vi "Init.vi"(4 "Data Queue Names":string[](array[string]), 6 "Data Notifier Names":string[](array[string]), 7 "Name":string, 8 "error in (no error)":errorcluster, 10 "MSS":refnum<class "Measure and Stimulus Subsystems.lvclass">, 11 "Sample PID Light in":refnum<class "Sample PID Light.lvclass">) -> (0 "error out":errorcluster, 3 "Sample PID Light out":refnum<class "Sample PID Light.lvclass">)   [LabVIEW 2023, in "Sample PID Light.lvclass"]
uses:
  Sample PID Light.lvclass
  Measure and Stimulus Subsystems/Measure and Stimulus Subsystems.lvclass
  Task/Task Base/Task Base.lvclass
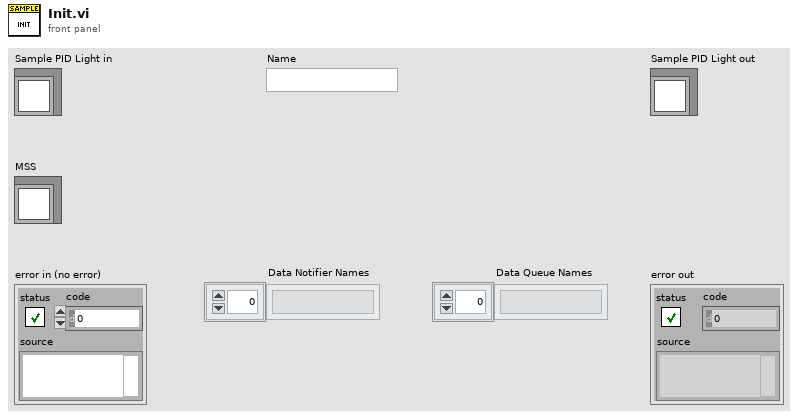
[diagram p1: front panel]
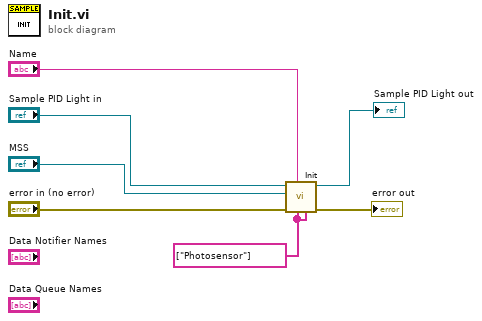
[diagram p0: block diagram]
diagram:
  w1 = string[] ["Photosensor"] ("Data Notifier Names")
  n1 = call-parent "Init.vi"("Data Queue Names"=w1, "Data Notifier Names"=w1, "Name"="Name", "error in (no error)"="error in (no error)", "MSS"="MSS", "Task Base in"="Sample PID Light in") -> ("error out"=→"error out":errorcluster, "Task Base out"=→"Sample PID Light out":refnum<class "Sample PID Light.lvclass">)  [unwired: 4 in]
